vi "IntializeDriveMotors.vi"() -> (7 "Left Motor Reference":T1, 8 "Right Motor Reference":T1)   [LabVIEW 2018]
uses:
  <vilib>/Rock Robotics/WPI/ThirdParty/Phoenix-LabVIEW/Motor Controller/Controls/CTRE_Phoenix_MotorControl_EnhancedMotorControllerConfigurables.ctl
  <vilib>/Rock Robotics/WPI/ThirdParty/Phoenix-LabVIEW/Motor Controller/Controls/CTRE_Phoenix_MotorControl_BaseConfigurables.ctl
  <vilib>/Rock Robotics/WPI/ThirdParty/Phoenix-LabVIEW/Motor Controller/Controls/CTRE_Phoenix_MotorControl_VelocityMeasurementPeriod.ctl
  <vilib>/Rock Robotics/WPI/ThirdParty/Phoenix-LabVIEW/Motor Controller/Controls/CTRE_Phoenix_MotorControl_SlotStructure.ctl
  <vilib>/Rock Robotics/WPI/ThirdParty/Phoenix-LabVIEW/Motor Controller/Controls/CTRE_Phoenix_MotorControl_FilterStruct.ctl
  <vilib>/Rock Robotics/WPI/ThirdParty/Phoenix-LabVIEW/Motor Controller/Controls/CTRE_Phoenix_MotorControl_RemoteSourceType.ctl
  <vilib>/Rock Robotics/WPI/ThirdParty/Phoenix-LabVIEW/Controls/CTRE_Phoenix_CustomParamConfiguration.ctl
  <vilib>/Rock Robotics/WPI/ThirdParty/Phoenix-LabVIEW/Motor Controller/Controls/CTRE_Phoenix_MotorControl_FeedbackDevice.ctl
  <vilib>/Rock Robotics/WPI/ThirdParty/Phoenix-LabVIEW/Motor Controller/Controls/CTRE_Phoenix_MotorControl_SensorTermFeedbackDevice_Enhanced.ctl
  <vilib>/Rock Robotics/WPI/ThirdParty/Phoenix-LabVIEW/Motor Controller/Controls/CTRE_Phoenix_MotorControl_LimitSwitchNormal.ctl
  <vilib>/Rock Robotics/WPI/ThirdParty/Phoenix-LabVIEW/Motor Controller/Controls/CTRE_Phoenix_MotorControl_LimitSwitchSource_Local.ctl
  <vilib>/Rock Robotics/WPI/MotorControl/WPI_MotorControlDeviceRef.ctl
  <vilib>/Rock Robotics/WPI/MotorControl/WPI_MotorControlType.ctl
  <vilib>/Rock Robotics/SystemInterfaces/DIO/FPGA_DIOPWMChannel.ctl
  <vilib>/Rock Robotics/WPI/PWM/WPI_PWMDeadband.ctl
  <vilib>/Rock Robotics/SystemInterfaces/DIO/FPGA_DIOChannel.ctl
panel:
  in  "Enhanced Motor Controller Configurables":T6={"Base Configurables"={"openLoopRamp"=0.0, "closedLoopRamp"=0.0, "peakOutputForward"=1.0, "peakOutputReverse"=-1.0, "nominalOutputForward"=0.0, "nominalOutputReverse"=0.0, "neutralDeadband"=0.04, "voltageCompSaturation"=0.0, "voltageMeasurementFilter"=32, "velocityMeasurementPeriod"=100, "velocityMeasurementWindow"=64, "forwardSoftLimitThreshold"=0, "reverseSoftLimitThreshold"=0, "forwardSoftLimitEnable"=FALSE, "reverseSoftLimitEnable"=FALSE, "slot0"={"P"=0.0, "I"=0.0, "D"=0.0, "F"=0.0, "integralZone"=0.0, "allowableClosedLoopError"=0, "maxIntegralAccumulator"=0.0, "closedLoopPeakOutput"=1.0, "closedLoopPeriod"=1}, "slot1"={"P"=0.0, "I"=0.0, "D"=0.0, "F"=0.0, "integralZone"=0.0, "allowableClosedLoopError"=0, "maxIntegralAccumulator"=0.0, "closedLoopPeakOutput"=1.0, "closedLoopPeriod"=1}, "slot2"={"P"=0.0, "I"=0.0, "D"=0.0, "F"=0.0, "integralZone"=0.0, "allowableClosedLoopError"=0, "maxIntegralAccumulator"=0.0, "closedLoopPeakOutput"=1.0, "closedLoopPeriod"=1}, "slot3"={"P"=0.0, "I"=0.0, "D"=0.0, "F"=0.0, "integralZone"=0.0, "allowableClosedLoopError"=0, "maxIntegralAccumulator"=0.0, "closedLoopPeakOutput"=1.0, "closedLoopPeriod"=1}, "auxPIDPolarity"=FALSE, "remoteFilter0"={"remoteSensorDeviceID"=0, "remoteSensorSource"=enum."Off"}, "remoteFilter1"={"remoteSensorDeviceID"=0, "remoteSensorSource"=enum."Off"}, "motionCruiseVelocity"=0, "motionAcceleration"=0, "motionProfileTrajectoryPeriod"=0, "feedbackNotContinuous"=FALSE, "remoteSensorClosedLoopDisableNeutralOnLOS"=FALSE, "clearPositionOnLimitF"=FALSE, "clearPositionOnLimitR"=FALSE, "clearPositionOnQuadIdx"=FALSE, "limitSwitchDisableNeutralOnLOS"=FALSE, "softLimitDisableNeutralOnLOS"=FALSE, "pulseWidthPeriod_EdgesPerRot"=1, "pulseWidthPeriod_FilterWindowSz"=1, "customParam"={"customParam0"=0, "customParam1"=0}, "trajectoryInterpolationEnable"=TRUE}, "primaryPID"={"selectedFeedbackCoefficient"=1.0, "selectedFeedbackSensor"=0}, "auxiliaryPID"={"selectedFeedbackCoefficient"=1.0, "selectedFeedbackSensor"=0}, "sum0Term"=0, "sum1Term"=0, "diff0Term"=0, "diff1Term"=0, "forwardLimitSwitchNormal"=enum."Normally Open", "reverseLimitSwitchNormal"=enum."Normally Open", "forwardLimitSwitchDeviceID"=0, "reverseLimitSwitchDeviceID"=0, "forwardLimitSwitchSource"=enum."Feedback Connector", "reverseLimitSwitchSource"=enum."Feedback Connector", "peakCurrentLimit"=1, "peakCurrentDuration"=1, "continuousCurrentLimit"=1} {"diff1Term" items=["QuadEncoder"=0, "Analog"=2, "Tachometer"=4, "Pulse Width Encoded Position"=8, "Remote Source 0"=11, "Remote Source 1"=12, "Software Emulated"=15]; "diff0Term" items=["QuadEncoder"=0, "Analog"=2, "Tachometer"=4, "Pulse Width Encoded Position"=8, "Remote Source 0"=11, "Remote Source 1"=12, "Software Emulated"=15]; "sum1Term" items=["QuadEncoder"=0, "Analog"=2, "Tachometer"=4, "Pulse Width Encoded Position"=8, "Remote Source 0"=11, "Remote Source 1"=12, "Software Emulated"=15]; "sum0Term" items=["QuadEncoder"=0, "Analog"=2, "Tachometer"=4, "Pulse Width Encoded Position"=8, "Remote Source 0"=11, "Remote Source 1"=12, "Software Emulated"=15]; "auxiliaryPID"."selectedFeedbackSensor" items=["QuadEncoder"=0, "Analog"=2, "Tachometer"=4, "Pulse Width Encoded Position"=8, "Sensor Sum (S0 + S1)"=9, "Sensor Difference (D0 - D1)"=10, "Remote Source 0"=11, "Remote Source 1"=12, "Software Emulated"=15]; "primaryPID"."selectedFeedbackSensor" items=["QuadEncoder"=0, "Analog"=2, "Tachometer"=4, "Pulse Width Encoded Position"=8, "Sensor Sum (S0 + S1)"=9, "Sensor Difference (D0 - D1)"=10, "Remote Source 0"=11, "Remote Source 1"=12, "Software Emulated"=15]; "Base Configurables"."velocityMeasurementPeriod" items=["Period_1ms"=1, "Period_2ms"=2, "Period_5ms"=5, "Period_10ms"=10, "Period_20ms"=20, "Period_25ms"=25, "Period_50ms"=50, "Period_100ms"=100]}
  # "Sum and Diff terms are ways to select more than one sensor as a feedback device. \n Sum 0 is the first feedback device to be used for the Sum term.\n Sum 1 is the feedback device to be added to Sum 0 for the Sum term.\n Diff 0 and Diff 1 work in a similar manner."
  # "These are only applicable\nif using a remote limit switch.\n\nLocal limit switches/no limit\nswitches do not use this."
  # "Current is below Continuous threshold AND\n\n(Requested output is weaker** than applied motor\noutput OR is in the opposite direction).\n/\nMotor output is set to requested output."
  # "Current is above Peak* Threshold for Peak Duration.\n/\nReduce motor output (towards neutral)."
  # "Current is below Continuous threshold.\n/\nRamp motor output towards requested output."
  # "Current is above Continuous threshold.\n/\nReduce motor output (towards neutral)."
  # "Current Limiting is NOT enabled\nby default.\nCall this VI to enable."
  # "*If the configured Peak Threshold is less than the Continuous Threshold, the applied Peak Threshold is set equal to the Configured Continuous Threshold in firmware.\n** Both requested output and applied motor output are in the same direction, and requested output is closer to neutral."
  # "False: Primary Output = PID[0] + PID[1]  ---  Auxiliary Output = PID[0] - PID[1]\nTrue:  Primary Output = PID[0] - PID[1] --- Auxiliary Output = PID[0] + PID[1]"
  # "Enable the motion profile executor to perform linear interpolation between profile points.  Defaults to True."
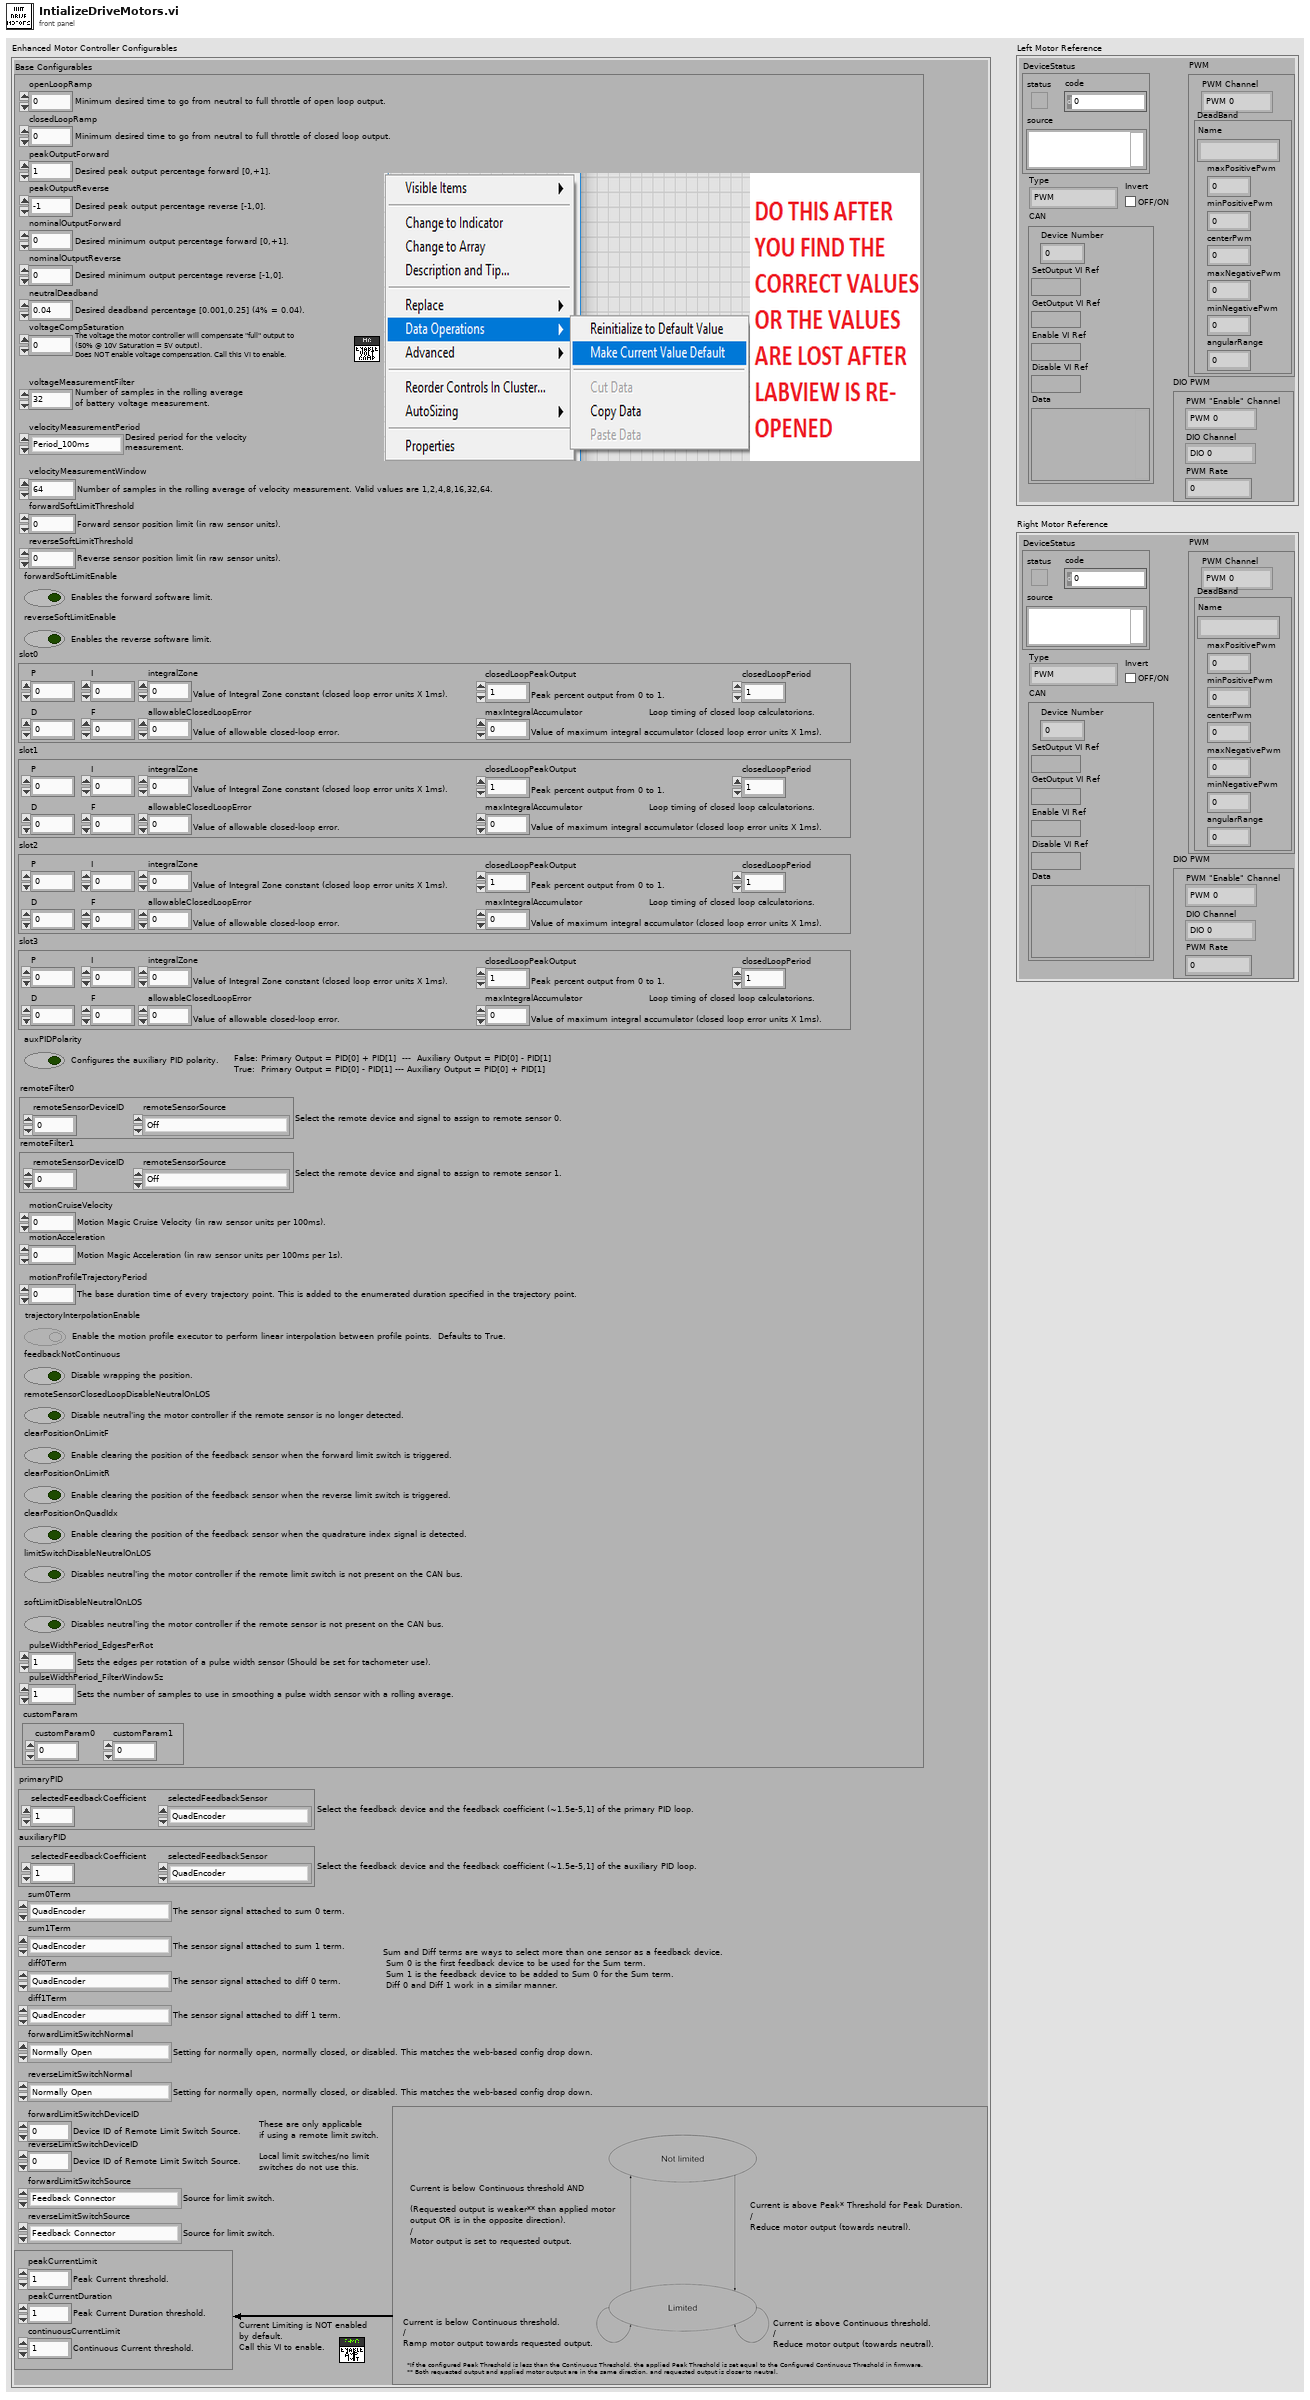
[diagram p1: front panel]
types:
  T1 = typedef "WPI_MotorControlDeviceRef.ctl" = cluster{"DeviceStatus":errorcluster, "Type":T2, "PWM":cluster{"PWM Channel":T3, "DeadBand":T4}, "CAN":cluster{"Device Number":u8, "SetOutput VI Ref":variant, "GetOutput VI Ref":variant, "Enable VI Ref":variant, "Disable VI Ref":variant, "Data":variant}, "Invert":bool, "DIO PWM":cluster{"PWM \"Enable\" Channel":T3, "DIOChannel":T5, "PWM Rate":dbl}}
  T2 = typedef "WPI_MotorControlType.ctl" = enum16{"PWM", "CAN", "DIO PWM"}
  T3 = typedef "FPGA_DIOPWMChannel.ctl" = enum8{"PWM 0", "PWM 1", "PWM 2", "PWM 3", "PWM 4", "PWM 5", "PWM 6", "PWM 7", "PWM 8", "PWM 9", "PWM MXP 0", "PWM MXP 1", "PWM MXP 2", "PWM MXP 3", "PWM MXP 4", "PWM MXP 5", "PWM MXP 6", "PWM MXP 7", "PWM MXP 8", "PWM MXP 9", "Invalid"}
  T4 = typedef "WPI_PWMDeadband.ctl" = cluster{"Name":string, "maxPositivePwm":i32, "minPositivePwm":i32, "centerPwm":i32, "maxNegativePwm":i32, "minNegativePwm":i32, "angularRange":u16}
  T5 = typedef "FPGA_DIOChannel.ctl" = enum8{"DIO 0", "DIO 1", "DIO 2", "DIO 3", "DIO 4", "DIO 5", "DIO 6", "DIO 7", "DIO 8", "DIO 9", "DIO MXP 0", "DIO MXP 1", "DIO MXP 2", "DIO MXP 3", "DIO MXP 4", "DIO MXP 5", "DIO MXP 6", "DIO MXP 7", "DIO MXP 8", "DIO MXP 9", "DIO MXP 10", "DIO MXP 11", "DIO MXP 12", "DIO MXP 13", "DIO MXP 14", "DIO MXP 15", "SPI Port CS1", "SPI Port CS2", "SPI Port CS3", "SPI Port MISO", "SPI Port MOSI", "Invalid"}
  T6 = typedef "CTRE_Phoenix_MotorControl_EnhancedMotorControllerConfigurables.ctl" = cluster{"Base Configurables":T7, "primaryPID":cluster{"selectedFeedbackCoefficient":dbl, "selectedFeedbackSensor":T13}, "auxiliaryPID":cluster{"selectedFeedbackCoefficient":dbl, "selectedFeedbackSensor":T13}, "sum0Term":T14, "sum1Term":T14, "diff0Term":T14, "diff1Term":T14, "forwardLimitSwitchNormal":T15, "reverseLimitSwitchNormal":T15, "forwardLimitSwitchDeviceID":i32, "reverseLimitSwitchDeviceID":i32, "forwardLimitSwitchSource":T16, "reverseLimitSwitchSource":T16, "peakCurrentLimit":i32, "peakCurrentDuration":i32, "continuousCurrentLimit":i32}
  T7 = typedef "CTRE_Phoenix_MotorControl_BaseConfigurables.ctl" = cluster{"openLoopRamp":dbl, "closedLoopRamp":dbl, "peakOutputForward":dbl, "peakOutputReverse":dbl, "nominalOutputForward":dbl, "nominalOutputReverse":dbl, "neutralDeadband":dbl, "voltageCompSaturation":dbl, "voltageMeasurementFilter":i32, "velocityMeasurementPeriod":T8, "velocityMeasurementWindow":i32, "forwardSoftLimitThreshold":i32, "reverseSoftLimitThreshold":i32, "forwardSoftLimitEnable":bool, "reverseSoftLimitEnable":bool, "slot0":T9, "slot1":T9, "slot2":T9, "slot3":T9, "auxPIDPolarity":bool, "remoteFilter0":T10, "remoteFilter1":T10, "motionCruiseVelocity":i32, "motionAcceleration":i32, "motionProfileTrajectoryPeriod":i32, "feedbackNotContinuous":bool, "remoteSensorClosedLoopDisableNeutralOnLOS":bool, "clearPositionOnLimitF":bool, "clearPositionOnLimitR":bool, "clearPositionOnQuadIdx":bool, "limitSwitchDisableNeutralOnLOS":bool, "softLimitDisableNeutralOnLOS":bool, "pulseWidthPeriod_EdgesPerRot":i32, "pulseWidthPeriod_FilterWindowSz":i32, "customParam":T12, "trajectoryInterpolationEnable":bool}
  T8 = typedef "CTRE_Phoenix_MotorControl_VelocityMeasurementPeriod.ctl" = u16
  T9 = typedef "CTRE_Phoenix_MotorControl_SlotStructure.ctl" = cluster{"P":dbl, "I":dbl, "D":dbl, "F":dbl, "integralZone":dbl, "allowableClosedLoopError":i32, "maxIntegralAccumulator":dbl, "closedLoopPeakOutput":dbl, "closedLoopPeriod":i32}
  T10 = typedef "CTRE_Phoenix_MotorControl_FilterStruct.ctl" = cluster{"remoteSensorDeviceID":u8, "remoteSensorSource":T11}
  T11 = typedef "CTRE_Phoenix_MotorControl_RemoteSourceType.ctl" = enum16{"Off", "Talon SRX Selected Sensor", "Pigeon IMU Yaw", "Pigeon IMU Pitch", "Pigeon IMU Roll", "CANifier Quadrature", "CANifier PWM Input 0", "CANifier PWM Input 1", "CANifier PWM Input 2", "CANifier PWM Input 3", "Gadgeteer Pigeon Yaw", "Gadgeteer Pigeon Pitch", "Gadgeteer Pigeon Roll"}
  T12 = typedef "CTRE_Phoenix_CustomParamConfiguration.ctl" = cluster{"customParam0":i32, "customParam1":i32}
  T13 = typedef "CTRE_Phoenix_MotorControl_FeedbackDevice.ctl" = i8
  T14 = typedef "CTRE_Phoenix_MotorControl_SensorTermFeedbackDevice_Enhanced.ctl" = i8
  T15 = typedef "CTRE_Phoenix_MotorControl_LimitSwitchNormal.ctl" = enum16{"Normally Open", "Normally Closed", "Disabled"}
  T16 = typedef "CTRE_Phoenix_MotorControl_LimitSwitchSource_Local.ctl" = enum16{"Feedback Connector", "Remote Talon SRX", "Remote CANifier", "Deactivated"}
  T17 = enum16{"FollowerType_PercentOutput", "FollowerType_AuxOutput1"}
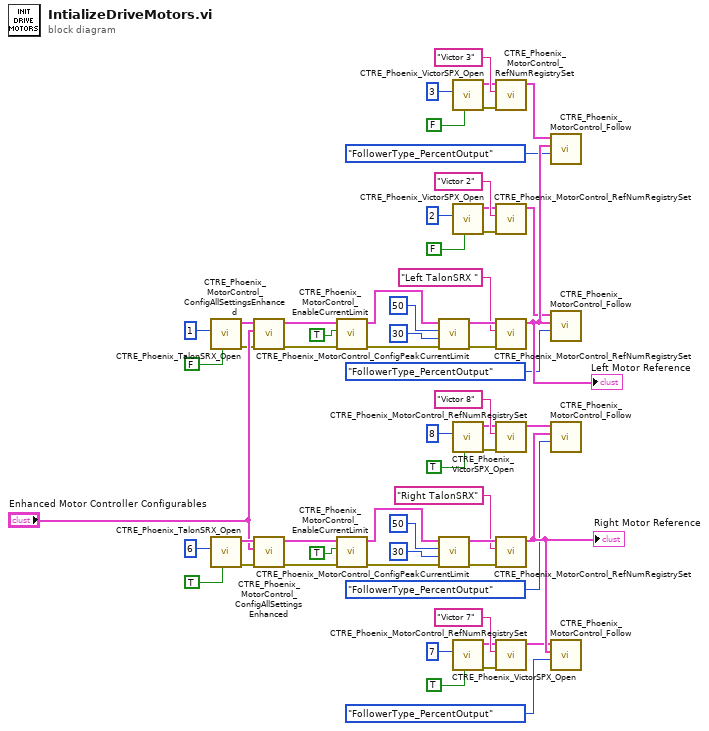
[diagram p0: block diagram]
diagram:
  n1 = call <vilib>:"CTRE_Phoenix_TalonSRX_Open.vi"("Invert"=FALSE, "Device Number"=u8 1) -> ("error out"=w23:errorcluster, "CAN Talon SRX Ref"=w24:T1)  [unwired: 8 in]
  n2 = call <vilib>:"CTRE_Phoenix_TalonSRX_Open.vi"("Invert"=TRUE, "Device Number"=u8 6) -> ("error out"=w27:errorcluster, "CAN Talon SRX Ref"=w26:T1)  [unwired: 8 in]
  n3 = call <vilib>:"CTRE_Phoenix_MotorControl_ConfigAllSettingsEnhanced.vi"("error in (no error)"=w23, "Enhanced Motor Controller Configurables"="Enhanced Motor Controller Configurables", "PhoenixMotorControlDevRef"=w24) -> ("error out"=w57:errorcluster, "PhoenixMotorControlDevRef"=w56:T1)  [unwired: 7 in]
  n4 = call <vilib>:"CTRE_Phoenix_MotorControl_ConfigAllSettingsEnhanced.vi"("error in (no error)"=w27, "Enhanced Motor Controller Configurables"="Enhanced Motor Controller Configurables", "PhoenixMotorControlDevRef"=w26) -> ("error out"=w48:errorcluster, "PhoenixMotorControlDevRef"=w47:T1)  [unwired: 7 in]
  n5 = call <vilib>:"CTRE_Phoenix_MotorControl_EnableCurrentLimit.vi"("error in (no error)"=w57, "Enable Current Limit?"=TRUE, "PhoenixMotorControlDevRef"=w56) -> ("error out"=w51:errorcluster, "PhoenixMotorControlDevRef"=w52:T1)  [unwired: 7 in]
  n6 = call <vilib>:"CTRE_Phoenix_MotorControl_EnableCurrentLimit.vi"("error in (no error)"=w48, "Enable Current Limit?"=TRUE, "PhoenixMotorControlDevRef"=w47) -> ("error out"=w42:errorcluster, "PhoenixMotorControlDevRef"=w43:T1)  [unwired: 7 in]
  n7 = call <vilib>:"CTRE_Phoenix_MotorControl_ConfigPeakCurrentLimit.vi"("error in (no error)"=w51, "Peak Current Maximum Duration (ms)"=30, "Peak Current (Amps)"=50, "PhoenixMotorControlDevRef"=w52) -> ("error out"=w58:errorcluster, "PhoenixMotorControlDevRef"=w59:T1)  [unwired: 6 in]
  n8 = call <vilib>:"CTRE_Phoenix_MotorControl_ConfigPeakCurrentLimit.vi"("error in (no error)"=w42, "Peak Current Maximum Duration (ms)"=30, "Peak Current (Amps)"=50, "PhoenixMotorControlDevRef"=w43) -> ("error out"=w50:errorcluster, "PhoenixMotorControlDevRef"=w49:T1)  [unwired: 6 in]
  n9 = call <vilib>:"CTRE_Phoenix_VictorSPX_Open.vi"("Invert"=FALSE, "Device Number"=u8 3) -> ("error out"=w8:errorcluster, "CAN Talon SRX Ref"=w7:T1)  [unwired: 8 in]
  n10 = call <vilib>:"CTRE_Phoenix_VictorSPX_Open.vi"("Invert"=FALSE, "Device Number"=u8 2) -> ("error out"=w4:errorcluster, "CAN Talon SRX Ref"=w3:T1)  [unwired: 8 in]
  n11 = call <vilib>:"CTRE_Phoenix_VictorSPX_Open.vi"("Invert"=TRUE, "Device Number"=u8 8) -> ("error out"=w5:errorcluster, "CAN Talon SRX Ref"=w6:T1)  [unwired: 8 in]
  n12 = call <vilib>:"CTRE_Phoenix_VictorSPX_Open.vi"("Invert"=TRUE, "Device Number"=u8 7) -> ("error out"=w9:errorcluster, "CAN Talon SRX Ref"=w10:T1)  [unwired: 8 in]
  n13 = call <vilib>:"CTRE_Phoenix_MotorControl_RefNumRegistrySet.vi"("error in (no error)"=w8, "refnum name"="Victor 3", "PhoenixMotorControlDevRef"=w7) -> ("PhoenixMotorControlDevRef"=w13:T1)  [unwired: 7 in, 1 out]
  n14 = call <vilib>:"CTRE_Phoenix_MotorControl_RefNumRegistrySet.vi"("error in (no error)"=w4, "refnum name"="Victor 2", "PhoenixMotorControlDevRef"=w3) -> ("PhoenixMotorControlDevRef"=w12:T1)  [unwired: 7 in, 1 out]
  n15 = call <vilib>:"CTRE_Phoenix_MotorControl_RefNumRegistrySet.vi"("error in (no error)"=w58, "refnum name"="Left TalonSRX ", "PhoenixMotorControlDevRef"=w59) -> ("PhoenixMotorControlDevRef"=w41:T1)  [unwired: 7 in, 1 out]
  "Left Motor Reference" <- w41
  n16 = call <vilib>:"CTRE_Phoenix_MotorControl_RefNumRegistrySet.vi"("error in (no error)"=w5, "refnum name"="Victor 8", "PhoenixMotorControlDevRef"=w6) -> ("PhoenixMotorControlDevRef"=w37:T1)  [unwired: 7 in, 1 out]
  n17 = call <vilib>:"CTRE_Phoenix_MotorControl_RefNumRegistrySet.vi"("error in (no error)"=w50, "refnum name"="Right TalonSRX", "PhoenixMotorControlDevRef"=w49) -> ("PhoenixMotorControlDevRef"=w40:T1)  [unwired: 7 in, 1 out]
  "Right Motor Reference" <- w40
  n18 = call <vilib>:"CTRE_Phoenix_MotorControl_RefNumRegistrySet.vi"("error in (no error)"=w9, "refnum name"="Victor 7", "PhoenixMotorControlDevRef"=w10) -> ("PhoenixMotorControlDevRef"=w35:T1)  [unwired: 7 in, 1 out]
  n19 = call <vilib>:"CTRE_Phoenix_MotorControl_Follow.vi"("FollowerType"=T17."FollowerType_PercentOutput", "Master Controller to Follow"=w41, "PhoenixMotorControlDevRef"=w13) -> ()  [unwired: 7 in, 2 out]
  n20 = call <vilib>:"CTRE_Phoenix_MotorControl_Follow.vi"("FollowerType"=T17."FollowerType_PercentOutput", "Master Controller to Follow"=w41, "PhoenixMotorControlDevRef"=w12) -> ()  [unwired: 7 in, 2 out]
  n21 = call <vilib>:"CTRE_Phoenix_MotorControl_Follow.vi"("FollowerType"=T17."FollowerType_PercentOutput", "Master Controller to Follow"=w40, "PhoenixMotorControlDevRef"=w37) -> ()  [unwired: 7 in, 2 out]
  n22 = call <vilib>:"CTRE_Phoenix_MotorControl_Follow.vi"("FollowerType"=T17."FollowerType_PercentOutput", "Master Controller to Follow"=w40, "PhoenixMotorControlDevRef"=w35) -> ()  [unwired: 7 in, 2 out]
